vi "E_reqs_by_time.vi"(8 "error_in":errorcluster, 9 "E_req":dbl[](array[numeric]), 10 "Data Model":T1={"Time_control"=[], "P_ch_av (from grid)"=[], "PV_exc (W)"=[], "PV_exc (Wh)"=[], "Delta_t"=0.0, "Timestamp"=0, "SOC_end (array)"=[], "SOC_ini (array)"=[], "SOC_max_min"=[], "N_periods"=0, "SOC_end"=[], "SOC_ini"=[], "t_end"=[], "t_ini"=[], "Plugged"=[], "P_charge vs. SOC"={"SOC"=[0.0, 100.0], "P"=[3700.0, 3700.0]}, "SOC_ini_save"=[], "SOC_ini_save (array)"=[]}, 11 "SOC_obj":dbl[](array[numeric])) -> (0 "error_out":errorcluster, 1 "SOC_values":dbl[][](array[numeric]), 2 "Plugged":i16[][](array[numeric]), 3 "Periods":i32[](array[numeric]))   [LabVIEW 2017]
uses:
  CONTROLS/Datamodel_FULL.ctl
  CONTROLS/P_ch_vs_SOC (array).ctl
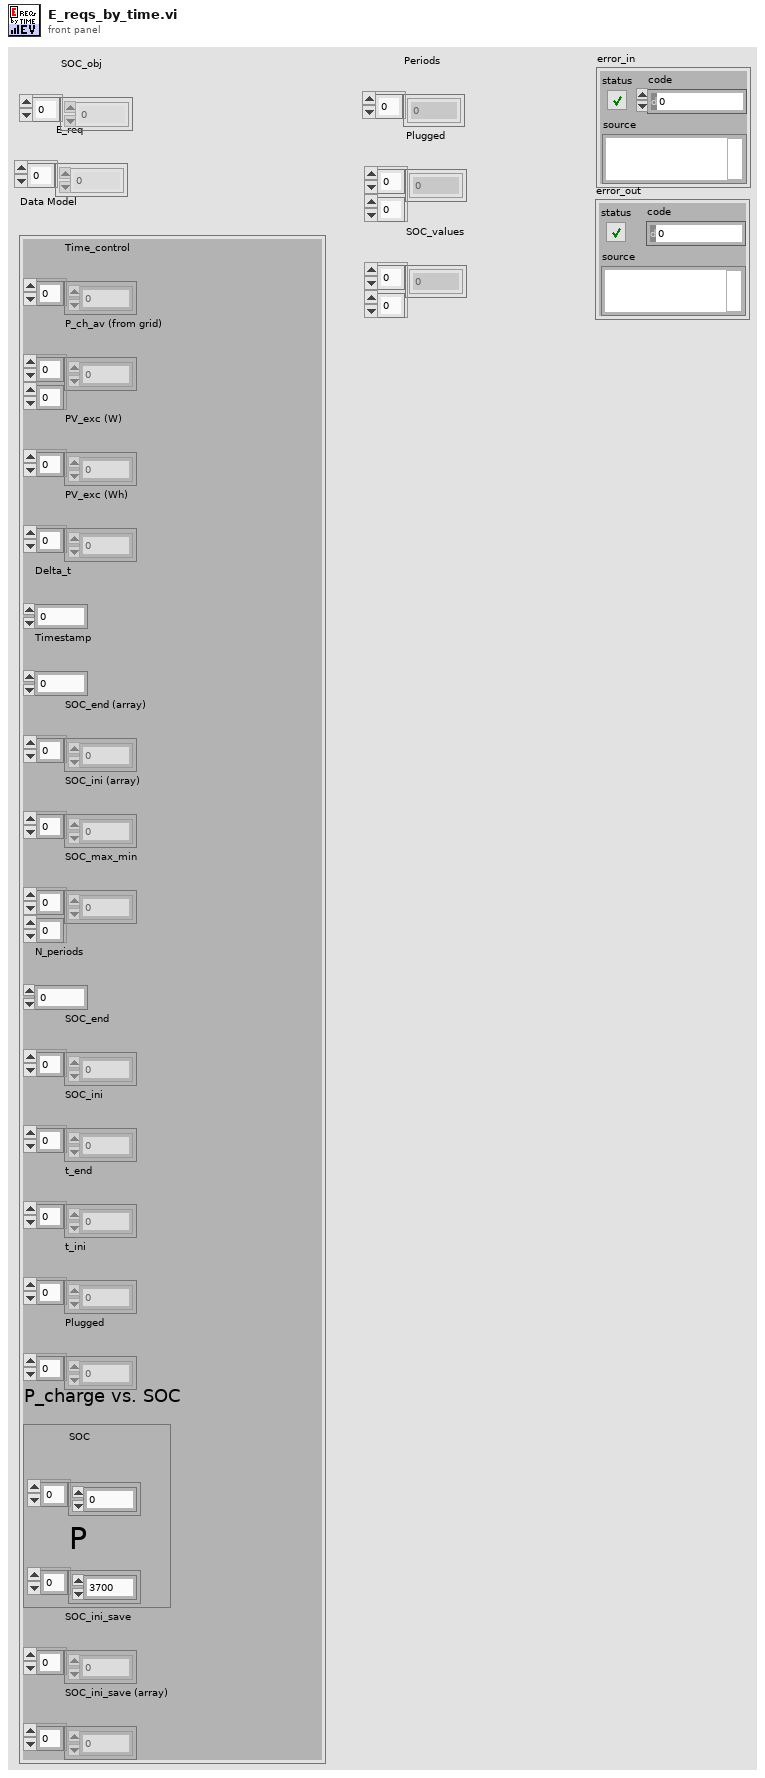
[diagram p1: front panel]
types:
  T1 = typedef "Datamodel_FULL.ctl" = cluster{"Time_control":i32[], "P_ch_av (from grid)":dbl[][], "PV_exc (W)":dbl[], "PV_exc (Wh)":dbl[], "Delta_t":dbl, "Timestamp":i32, "SOC_end (array)":dbl[], "SOC_ini (array)":dbl[], "SOC_max_min":dbl[][], "N_periods":i32, "SOC_end":dbl[], "SOC_ini":dbl[], "t_end":i32[], "t_ini":i32[], "Plugged":i32[], "P_charge vs. SOC":T2, "SOC_ini_save":dbl[], "SOC_ini_save (array)":dbl[]}
  T2 = typedef "P_ch_vs_SOC (array).ctl" = cluster{"SOC":dbl[], "P":dbl[]}
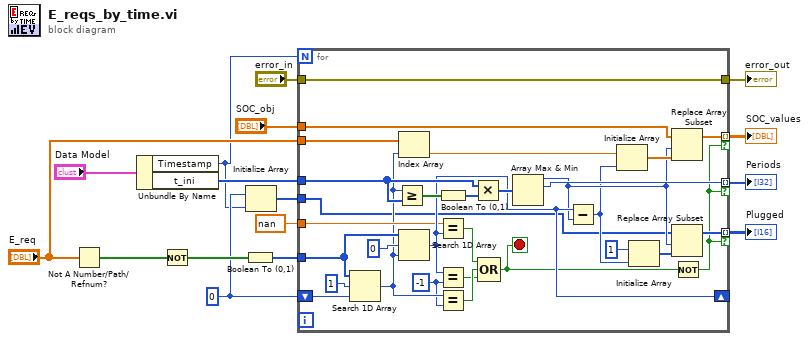
[diagram p0: block diagram]
diagram:
  w6 = 0
  n1 = Not A Number/Path/Refnum?(number/path/refnum="E_req") -> (NaN/Path/Refnum?=w8:bool[])
  n2 = Unbundle By Name("Data Model") -> ("Timestamp"=w1:i32, "t_ini"=w10:i32[])
  n3 = Not(x=w8) -> (.not. x?=w7:bool[])
  n4 = Boolean To (0,1)(Boolean=w7) -> (0, 1=w16:i16[])
  n5 = Initialize Array(w6, w1) -> (w5:i32[])
  n6 = for {
    N: w1 -> [_]
    tunnel: w16 -> [w44]
    tunnel: [w41] -> w15 mode=indexing if=w20
    tunnel: "SOC_obj" -> [w26]
    shift-right: [w35] -> _
    shift-left: w6 -> [w36]
    tunnel: w10 -> [w38]
    tunnel: nan -> [w34]
    tunnel: [w30] -> w14 mode=indexing if=w20
    tunnel: [w27] -> w12 mode=indexing if=w20
    tunnel: "E_req" -> [w25]
    tunnel: w5 -> [w19]
    tunnel: [w18] -> w3
    tunnel: "error_in" -> [w18]
    stop <- w21 stop-if-true
    w17 = i16 -1 ("element")
    n7 = Search 1D Array(1D array=w44, element=i16 1, start index (0)=w36) -> (index of element=w24:i32)
    n8 = Greater Or Equal?(x=w24, y=w38) -> (x >= y?=w40:bool[])
    n9 = Index Array(array=w25, index=w24) -> (element=w23:dbl)
    n10 = Search 1D Array(1D array=w44, element=i16 0, start index (0)=w24) -> (index of element=w35:i32)
    n11 = Boolean To (0,1)(Boolean=w40) -> (0, 1=w39:i16[])
    n12 = Equal?(x=w34, y=w35) -> (x = y?=w33:bool)
    n13 = Equal?(x=w35, y=w17) -> (x = y?=w31:bool)
    n14 = Equal?(x=w24, y=w17) -> (x = y?=w32:bool)
    n15 = Multiply(x=w38, y=w39) -> (x*y=w37:i32[])
    n16 = Compound Arithmetic op=OR(w33, w32, w31) -> (w21:bool)
    n17 = Array Max & Min(array=w37) -> (max value=w28:i32, max index (indices)=w30:i32)  [unwired: 2 out]
    n18 = Subtract(x=w35, y=w28) -> (x-y=w22:i32)
    n19 = Initialize Array(w23, w22) -> (w29:dbl[])
    n20 = Initialize Array(i16 1 ("element"), w22) -> (w42:i16[])
    n21 = Replace Array Subset(array=w26, new element=w29, index=w28) -> (w27:dbl[])
    n22 = Replace Array Subset(array=w19, new element=w42, index=w28) -> (w41:i32[])
    n23 = Not(x=w21) -> (.not. x?=w20:bool)
  }
  "Plugged" <- w15
  "Periods" <- w14
  "SOC_values" <- w12
  "error_out" <- w3
